vi "PH_AxisGUI_BaseClass.ReadDB.vi"(0 "i ref in":refnum<vi>, 5 "error in (no error)":errorcluster) -> (14 "i ref out":refnum<vi>, 15 "Address Axis 1":T1={"Instance"="N/A", "Motor Nr"=0}, 16 "Address Axis 2":T1={"Instance"="N/A", "Motor Nr"=0} caption="element", 17 "Name Axis 1":string, 18 "Name Axis 2":string, 19 "error out":errorcluster)   [LabVIEW 2014]
doc: "This VI reads the DB special 0 and 1 DB entries which are the axis names and writes them to own attributes. Depending on this, several GUI elements are set."
uses:
  PH_Common/PH_Motion/PH_Motion.Axis Address.ctl
  CSCore/BaseProcess/BaseProcess.lvlib
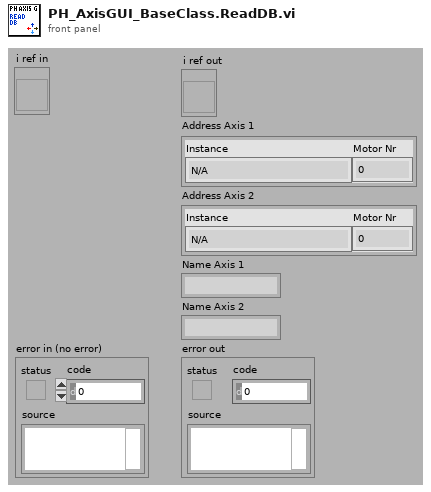
[diagram p1: front panel]
types:
  T1 = typedef "PH_Motion.Axis Address.ctl" = cluster{"Instance":string, "Motor Nr":i32}
  T2 = typedef "BaseProcess.lvlib/BaseProcess.i attribute.ctl" = cluster{"EventStatus":string, "EventError":i32, "PresetEvtWatchD":i32, "PresetPdcWatchD":i32, "EventTimeout":i32, "PeriodicInterval":i32, "Interface":string[], "Address":string[], "Special":string[], "PeriodicError":i32, "PeriodicStatus":string, "SuperProc":string, "Descriptors":T3[], "CaseRef":refnum<vi>, "PdcRef":refnum<vi>, "Thread Ref":refnum<vi>, "eventErrorID":i32, "eventStatusID":i32, "periodicErrorID":i32, "periodicStatusID":i32, "pdcCtrID":i32}
  T3 = typedef "BaseProcess.lvlib/BaseProcess.descriptor definition.ctl" = cluster{"selector":string, "descriptor":T4}
  T4 = typedef "BaseProcess.lvlib/BaseProcess.descriptor string definition.ctl" = string
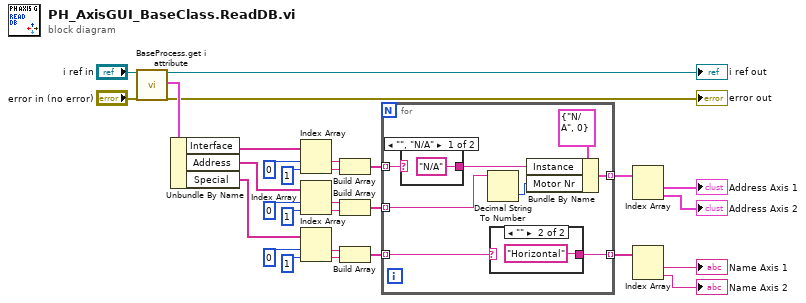
[diagram p0: block diagram]
diagram:
  n1 = call "BaseProcess.get i attribute.vi"("i ref in"="i ref in", "error in (no error)"="error in (no error)") -> ("i ref out"=→"i ref out":refnum<vi>, "i attribute"=w27:T2, "error out"=→"error out":errorcluster)  [unwired: 15 in]
  n2 = Unbundle By Name(w27) -> ("Interface"=w26:string[], "Address"=w18:string[], "Special"=w9:string[])
  n3 = Index Array(array=w26, index #1=0 ("index"), index #2=1 ("index")) -> (element #1=w23:string, element #2=w22:string)
  n4 = Index Array(array=w18, index #1=0 ("index"), index #2=1 ("index")) -> (element #1=w17:string, element #2=w14:string)
  n5 = Index Array(array=w9, index #1=0 ("index"), index #2=1 ("index")) -> (element #1=w12:string, element #2=w11:string)
  n6 = Build Array(w23, w22) -> (w21:string[])
  n7 = Build Array(w17, w14) -> (w13:string[])
  n8 = Build Array(w12, w11) -> (w10:string[])
  n9 = for {
    tunnel: w21 -> [w31] mode=indexing
    tunnel: w13 -> [w35] mode=indexing
    tunnel: w10 -> [w33] mode=indexing
    tunnel: [w36] -> w8 mode=indexing
    tunnel: [w32] -> w5 mode=indexing
    n10 = case shown="\"\", \"N/A\"" w31 {
      selector: w31 -> [_ w39]
      tunnel: ["N/A" w39] -> w30
      frame "", "N/A" {
      }
      frame Default {
      }
    }
    n11 = Decimal String To Number(string=w35) -> (number=w34:i32)  [unwired: 2 in, 1 out]
    n12 = case shown="\"\"" w33 {
      selector: w33 -> [w40 _]
      tunnel: [w40 "Horizontal"] -> w32
      frame Default {
      }
      frame "" {
      }
    }
    n13 = Bundle By Name(cluster=T1 {"Instance"="N/A", "Motor Nr"=0} ("Axis1_Information"), "Instance"=w30, "Motor Nr"=w34) -> (w36:T1)
  }
  n14 = Index Array(array=w8) -> (element #1=→"Address Axis 1":T1, element #2=→"Address Axis 2":T1)  [unwired: 2 in]
  n15 = Index Array(array=w5) -> (element #1=→"Name Axis 1":string, element #2=→"Name Axis 2":string)  [unwired: 2 in]
